vi "Create Map of tokens to replace.vi"() -> (3 "Tokens to replace":map{string, string}(c390))   [LabVIEW 2020, in "ConstantErrorsMaker.lvlib"]
uses:
  ConstantErrorsMaker.lvlib
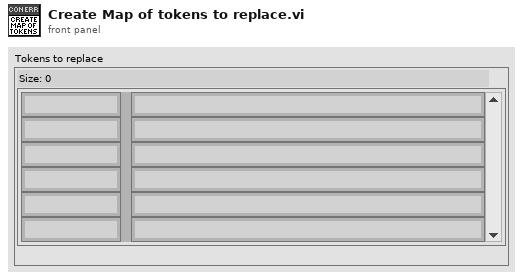
[diagram p1: front panel]
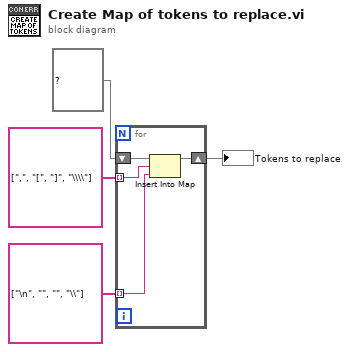
[diagram p0: block diagram]
diagram:
  n1 = for {
    shift-right: [w7] -> w4
    shift-left: map{string, string} {} ("Tokens to replace") -> [w8]
    tunnel: string[] [",", "[", "]", "\\\\"] -> [w6] mode=indexing
    tunnel: string[] ["\n", "", "", "\\"] -> [w5] mode=indexing
    n2 = Insert Into Map(map in=w8, key=w6, value=w5) -> (map out=w7:map{string, string})  [unwired: 2 out]
  }
  "Tokens to replace" <- w4
